vi "GetMultiAiChans.vi"(8 "TimeOut (ms)":i32=1000, 9 "ChansSel":T1, 10 "Num":u32=1000 caption="PtsToRead", 11 "error in":errorcluster caption="错误输入") -> (0 "Data":sgl[][](array[numeric]), 3 "error out":errorcluster caption="错误输出")   [LabVIEW 2016]
uses:
  PLC-Lab/lib/gusb.dll
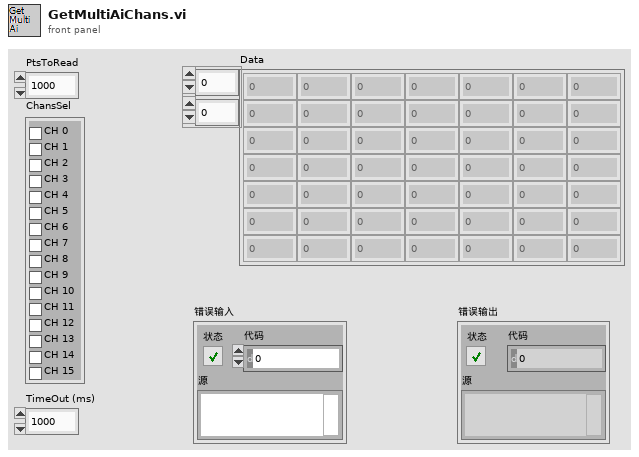
[diagram p1: front panel]
types:
  T1 = cluster{"CH 0":bool, "CH 1":bool, "CH 2":bool, "CH 3":bool, "CH 4":bool, "CH 5":bool, "CH 6":bool, "CH 7":bool, "CH 8":bool, "CH 9":bool, "CH 10":bool, "CH 11":bool, "CH 12":bool, "CH 13":bool, "CH 14":bool, "CH 15":bool}
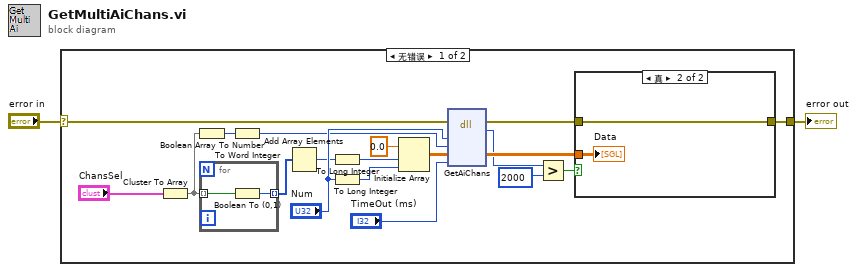
[diagram p0: block diagram]
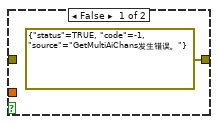
[diagram p2: hidden frame]
diagram:
  n1 = case shown="无错误" "error in" {
    selector: "error in" -> [w20 w27]
    tunnel: [w3 w27] -> w1
    frame No Error {
      n2 = Cluster To Array(cluster="ChansSel") -> (array=w13:bool[])
      n3 = Boolean Array To Number(Boolean array=w13) -> (number=w15:u32)
      n4 = for {
        tunnel: w13 -> [w26] mode=indexing
        tunnel: [w25] -> w12 mode=indexing
        n5 = Boolean To (0,1)(Boolean=w26) -> (0, 1=w25:i16)
      }
      n6 = To Word Integer(number=w15) -> (16bit integer=w14:i16)
      n7 = Add Array Elements(numeric array=w12) -> (sum=w11:i16)
      n8 = To Long Integer(number=w11) -> (32bit integer=w10:i32)
      n9 = To Long Integer(number="Num") -> (32bit integer=w19:i32)
      n10 = Initialize Array(sgl 0.0 ("元素"), w10, w19) -> (w9:sgl[][])
      n11 = dll-call lib="E:/Camproject/2018/2018.1Labview/PLC-Lab/lib/gusb.dll" fn="GetAiChans"(error in=w20, "Num"="Num", "ChanSel"=w14, "Buf"=w9, "TimeOut"="TimeOut (ms)") -> (error out=w4:errorcluster, "Status"=w7:i32, "Buf"=w8:sgl[][])  [unwired: 5 in, 1 out]
      n12 = Greater?(x=w7, y=2000) -> (0:w5:bool)
      n13 = case shown="真" w5 {
        tunnel: [errorcluster {"status"=TRUE, "code"=-1, "source"="GetMultiAiChans发生错误。"} ("错误常量") w24] -> w3
        tunnel: w4 -> [_ w24]
        tunnel: w8 -> [_ w23]
        frame False {
        }
        frame True {
          "Data" <- w23
        }
      }
    }
    frame Error {
    }
  }
  "error out" <- w1
